vi "Construct Slave Config.vi"(8 "error in (no error)":errorcluster, 11 "Function in":refnum<class "Function.lvclass">) -> (0 "error out":errorcluster, 3 "Function out":refnum<class "Function.lvclass">)   [LabVIEW 2016, in "Function Actor.lvlib" / "Function.lvclass"]
uses:
  <userlib>/Common Components/Function Actor/Function.lvclass
  <userlib>/Common Components/Slave Configuration/Slave Config.lvclass
  C:/Program Files (x86)/National Instruments/LabVIEW 2016/user.lib/Configuration Dialog Actor/Configuration.lvclass
  <userlib>/Common Components/Function Actor/Function.lvclass/Function.ctl
  <userlib>/Common Components/Slave Configuration/Slave Config.lvclass/Slave Config.ctl
  <userlib>/Common Components/Function Actor/Accessors/Read TCP Connection Info.vi
  <userlib>/Common Components/Slave Configuration/Config/Read IP Address of Server.vi
  <userlib>/Common Components/Slave Configuration/Config/Read remote port.vi
  <userlib>/Common Components/Function Actor/Accessors/Write TCP Connection Info.vi
  <userlib>/Configuration Dialog Actor/Configuration.lvclass
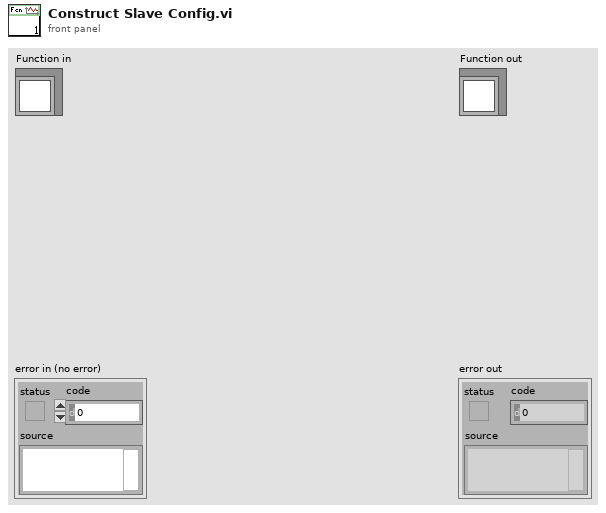
[diagram p1: front panel]
types:
  T1 = enum16{"open", "replace", "create", "open or create", "replace or create", "replace or create with confirmation"}
  T2 = typedef "Function Actor.lvlib/Function.lvclass/TCP connection info.ctl" = cluster{"Server Address":string, "Port":u16, "Timeout (ms)":i32, "Retry-interval (ms)":i32}
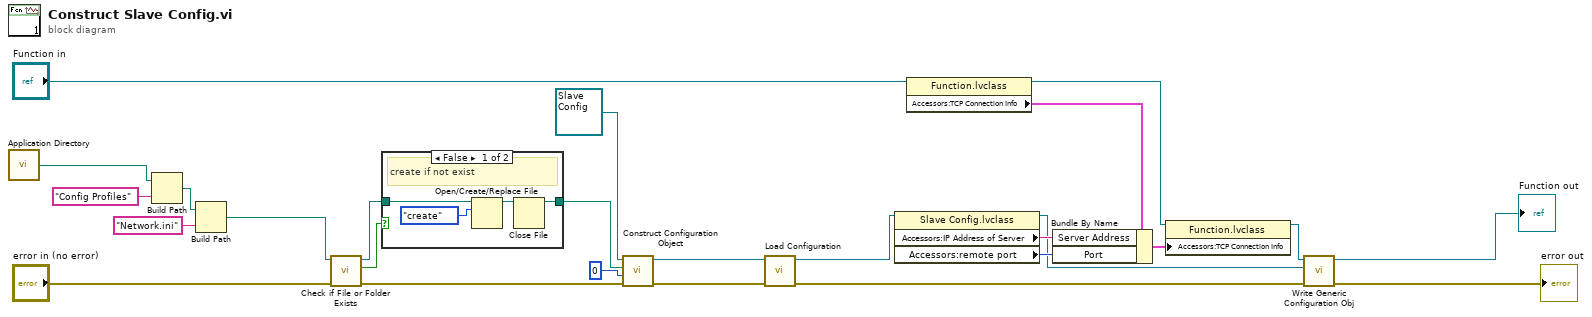
[diagram p0: block diagram]
diagram:
  n1 = call <vilib>:"Application Directory.vi"() -> ("Application Directory"=w25:path)
  n2 = Build Path(base path=w25, name or relative path="Config Profiles") -> (appended path=w22:path)
  n3 = Build Path(base path=w22, name or relative path="Network.ini") -> (appended path=w24:path)
  n4 = call <vilib>:"Check if File or Folder Exists.vi"("error in (no error)"="error in (no error)", "path"=w24) -> ("error out"=w4:errorcluster, "file or folder exists?"=w21:bool, "dup path"=w23:path)  [unwired: 7 in]
  n5 = case shown="False" w21 {
    tunnel: w23 -> [w30 w31]
    tunnel: [w27 w31] -> w11
    frame False {
      # "create if not exist"
      n6 = Open/Create/Replace File(file path (use dialog)=w30, operation (0:open)=T1."create") -> (refnum out=w28:refnum<file>)  [unwired: 4 in, 2 out]
      n7 = Close File(refnum=w28) -> (path=w27:path)  [unwired: 1 in, 1 out]
    }
    frame True {
    }
  }
  n8 = call <userlib>:"Construct Configuration Object.vi"("error in (no error)"=w4, "Initial Category Selection"=0, "Configuration File Path"=w11, "Configuration in"=refnum<class "Slave Config.lvclass"> refnum ("Slave Config.lvclass")) -> ("error out"=w3:errorcluster, "Configuration out"=w17:refnum<class "Slave Config.lvclass">)  [unwired: 4 in, 2 out]
  n9 = call <userlib>:"Load Configuration.vi"("error in (no error)"=w3, "Configuration in"=w17) -> ("error out"=w2:errorcluster, "Configuration out"=w16:refnum<class "Slave Config.lvclass">)  [unwired: 7 in, 1 out]
  n10 = property class="Slave Config.lvclass"(reference=w16) -> (reference out=w6:refnum<class "Slave Config.lvclass">, "Accessors:IP Address of Server"=w14:string, "Accessors:remote port"=w13:u16)  [unwired: 1 in, 1 out]
  n11 = property class="Function.lvclass"(reference="Function in") -> (reference out=w9:refnum<class "Function.lvclass">, "Accessors:TCP Connection Info"=w15:T2)  [unwired: 1 in, 1 out]
  n12 = Bundle By Name(cluster=w15, "Server Address"=w14, "Port"=w13) -> (w12:T2)
  n13 = property class="Function.lvclass"(reference=w9, "Accessors:TCP Connection Info"=w12) -> (reference out=w8:refnum<class "Function.lvclass">)  [unwired: 1 in, 1 out]
  n14 = call <userlib>:"Write Generic Configuration Obj.vi"("error in (no error)"=w2, "Configuration.lvlib:Configuration.lvclass"=w6, "Function in"=w8) -> ("error out"=→"error out":errorcluster, "Function out"=→"Function out":refnum<class "Function.lvclass">)  [unwired: 7 in]
